vi "CmdExe.ExecCmd with Timeout and Abort_V2.vi"(0 "Working Dir":path=path "", 1 "Run minimized? (T)":bool=TRUE, 2 "Wait until completion? (T)":bool=TRUE, 3 "IgnoreStdErr":bool, 5 "Executable":string, 7 "StdIn":string, 9 "Arguements":string, 11 "error in":errorcluster, 12 "Timeout ms(-1)":i32=-1) -> (4 "STD OUT":string, 6 "STD ERR":string, 10 "Timed Out":bool, 13 "Aborted":bool, 14 "return code":i32, 15 "error out":errorcluster)   [LabVIEW 2024]
panel:
  out "Task Killed":bool
  # "Launch Cmd Exe"
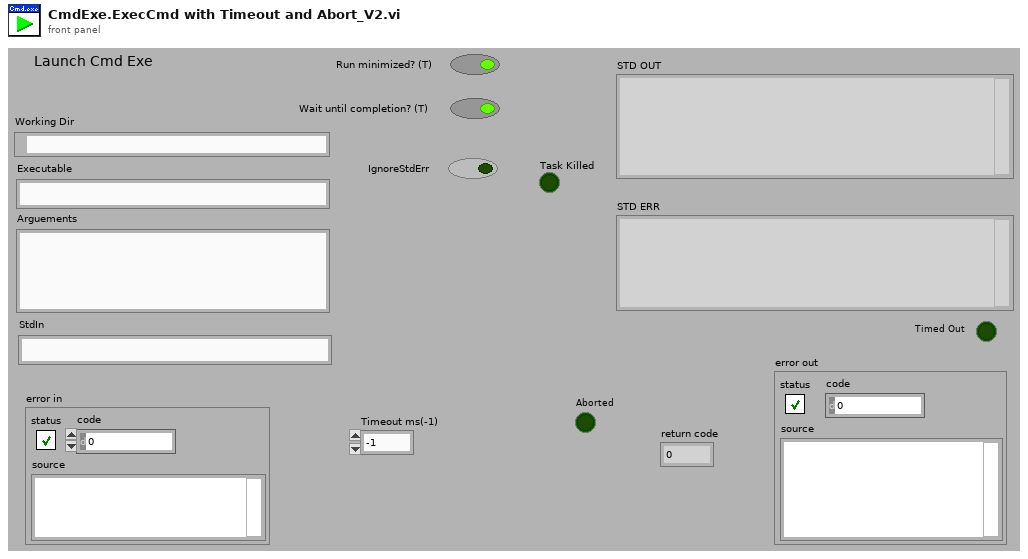
[diagram p1: front panel]
types:
  T1 = cluster{"Ref":refnum<vi>, "Abort":bool, "Timeout":bool, "Cmd":string, "Exe":string, "StdErr":string}
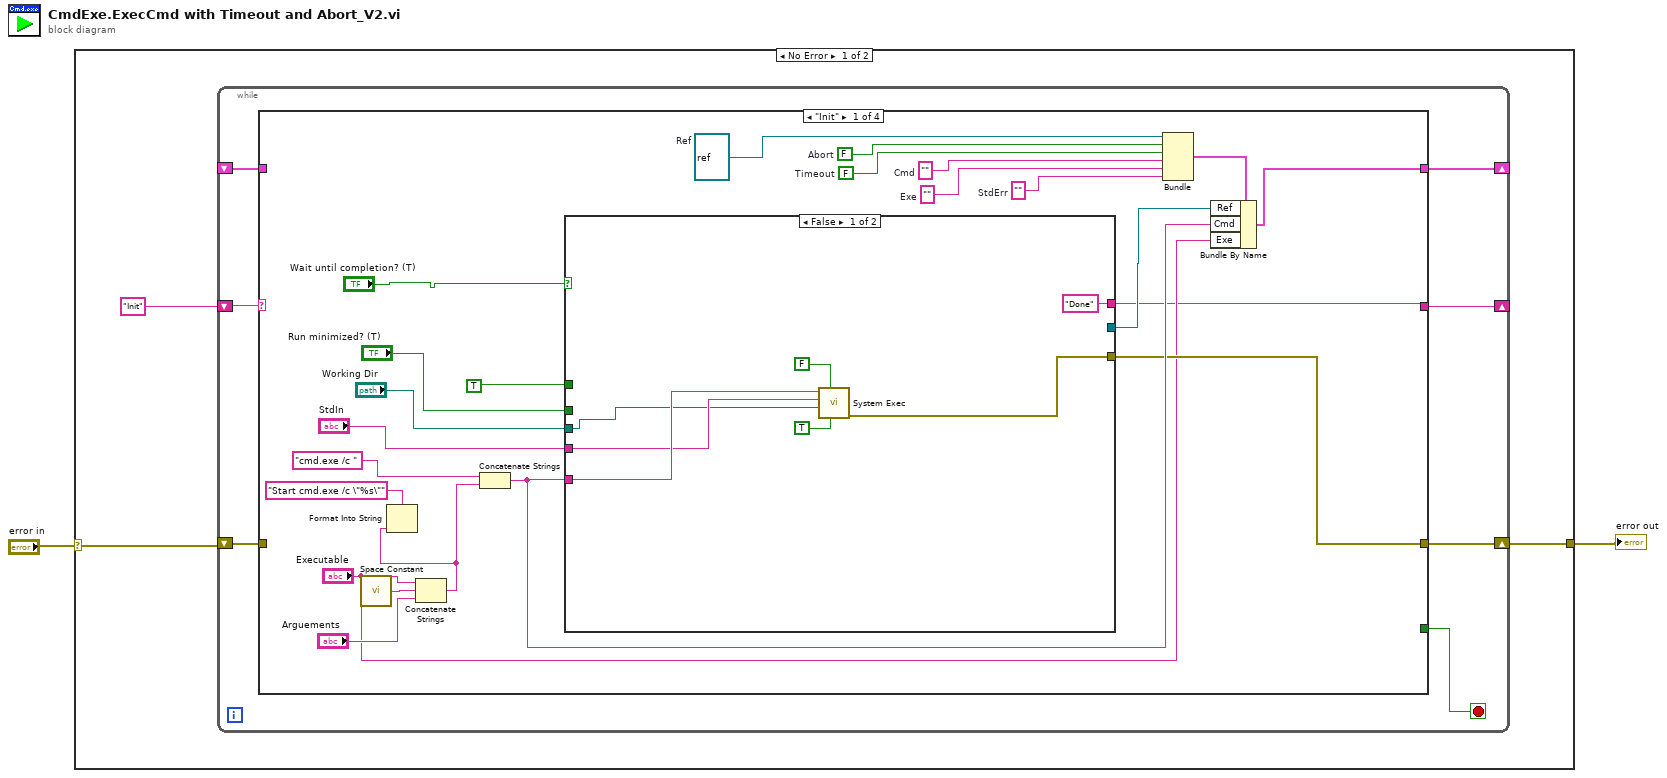
[diagram p0: block diagram]
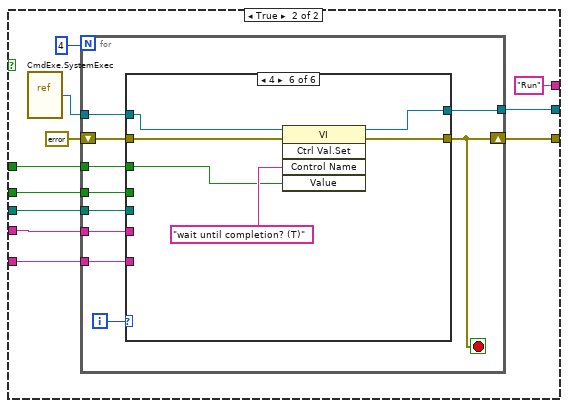
[diagram p2: hidden frame]
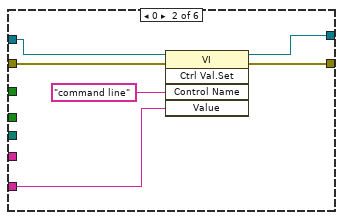
[diagram p4: hidden frame]
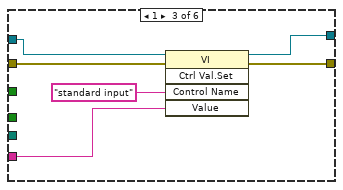
[diagram p5: hidden frame]
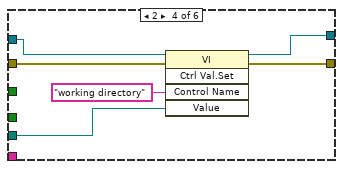
[diagram p6: hidden frame]
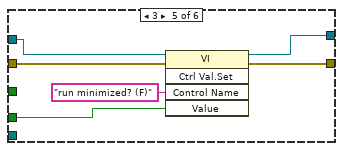
[diagram p7: hidden frame]
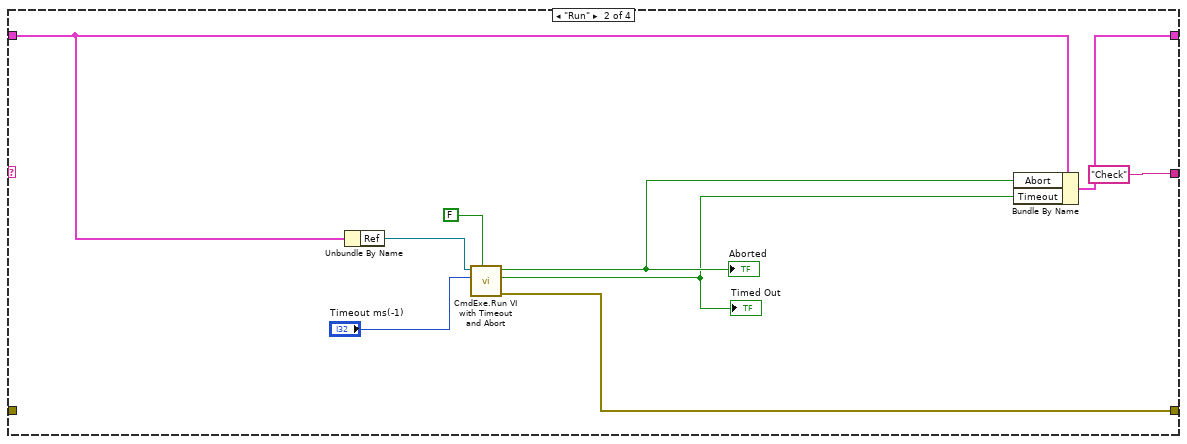
[diagram p8: hidden frame]
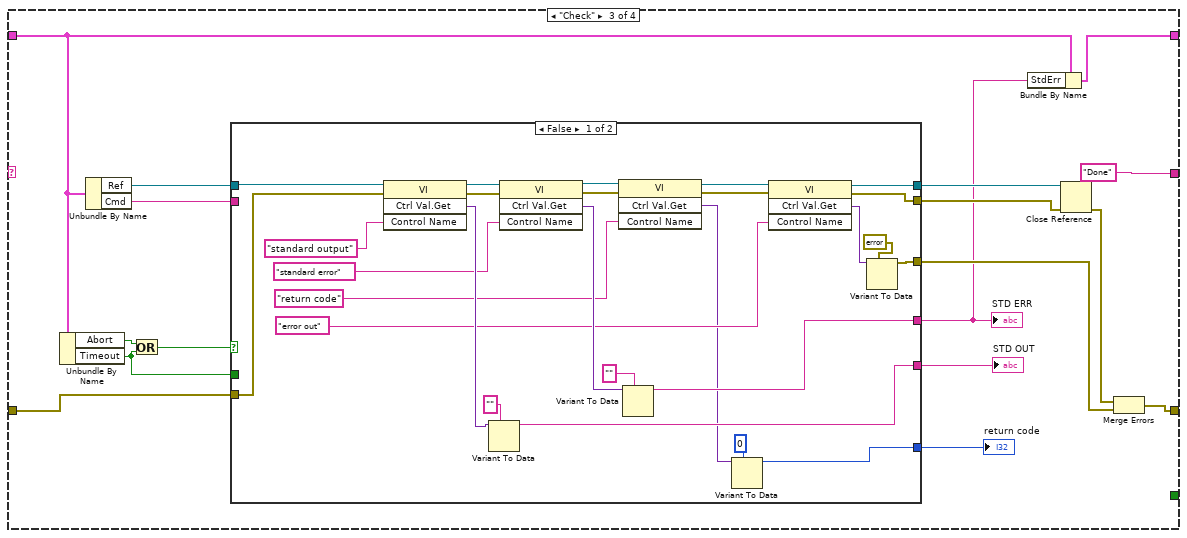
[diagram p9: hidden frame]
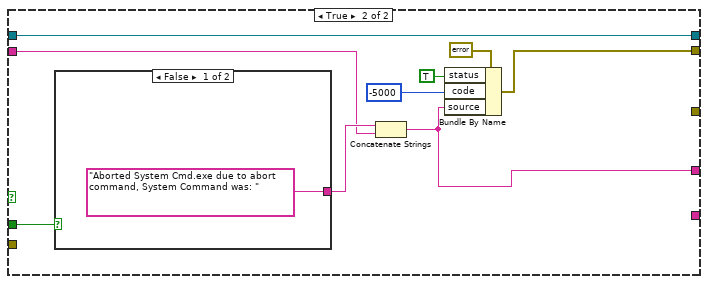
[diagram p10: hidden frame]
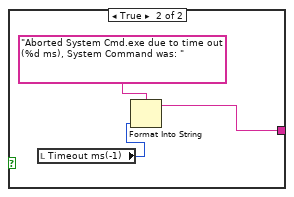
[diagram p11: hidden frame]
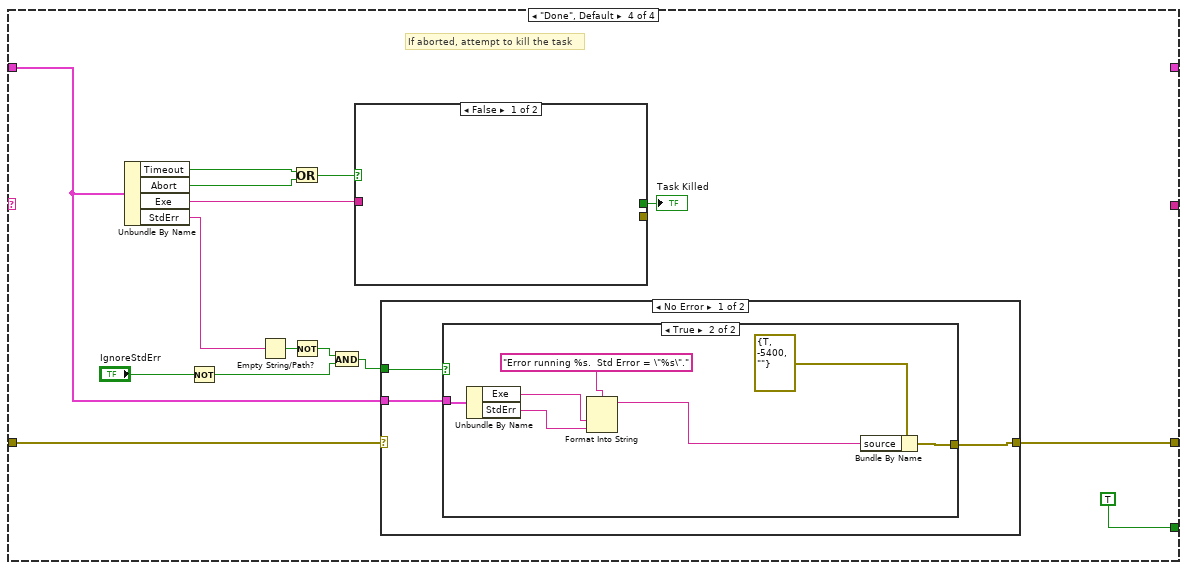
[diagram p12: hidden frame]
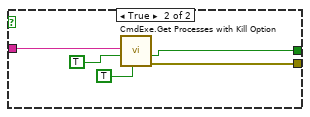
[diagram p15: hidden frame]
diagram:
  n1 = case shown="No Error" "error in" {
    selector: "error in" -> [w4 w192]
    tunnel: [w3 w192] -> w1
    frame No Error {
      n2 = while {
        shift-right: [w10] -> _
        shift-left: _ -> [w11]
        shift-right: [w9] -> _
        shift-left: "Init" -> [w12]
        shift-right: [w7] -> w3
        shift-left: w4 -> [w8]
        stop <- w6 stop-if-true
        n3 = case shown="\"Init\"" w12 {
          tunnel: w11 -> [_ w102 w108 w166]
          tunnel: [w29 w101 w107 _] -> w10
          tunnel: [w17 "Check" "Done" _] -> w9
          tunnel: [_ _ _ TRUE] -> w6
          tunnel: w8 -> [_ _ w113 w169]
          tunnel: [w24 w98 w111 w167] -> w7
          frame "Init" {
            w19 = ""  # StdErr
            w21 = ""  # Exe
            w26 = ""  # Cmd
            w27 = FALSE  # Timeout
            w28 = FALSE  # Abort
            w32 = refnum<vi> refnum  # Ref
            n4 = call <vilib>:"Space Constant.vi"() -> ("String"=w22:string)
            n5 = Concatenate Strings("Executable", w22, "Arguements") -> (w13:string)
            n6 = Format Into String(format string="Start cmd.exe /c \"%s\"", w13) -> ()  [unwired: 2 in, 2 out]
            n7 = Concatenate Strings("cmd.exe /c ", w13) -> (w25:string)
            n8 = case shown="False" "Wait until completion? (T)" {
              tunnel: "Run minimized? (T)" -> [_ w53]
              tunnel: "Working Dir" -> [w39 w52]
              tunnel: [_ w51] -> w31
              tunnel: w25 -> [w41 w50]
              tunnel: [w37 w49] -> w24
              tunnel: "StdIn" -> [w40 w48]
              tunnel: ["Done" "Run"] -> w17
              tunnel: TRUE -> [_ w43]
              frame False {
                n9 = call <vilib>:"System Exec.vi"("run minimized? (F)"=TRUE, "wait until completion? (T)"=FALSE, "working directory"=w39, "standard input"=w40, "command line"=w41) -> ("error out"=w37:errorcluster)  [unwired: 3 in, 3 out]
              }
              frame True {
                n10 = vi-ref "CmdExe.SystemExec.vi"() -> (w46:refnum<vi>)
                n11 = for {
                  N: 4 -> [_]
                  shift-right: [w54] -> w49
                  shift-left: errorcluster {"status"=FALSE, "code"=0, "source"=""} ("error constant") -> [w63]
                  tunnel: w46 -> [w62]
                  tunnel: [w61] -> w51
                  tunnel: w50 -> [w59]
                  tunnel: w48 -> [w58]
                  tunnel: w52 -> [w57]
                  tunnel: w53 -> [w56]
                  tunnel: w43 -> [w55]
                  i -> [w60]
                  stop <- w54 stop-if-true
                  n12 = case shown="4" w60 {
                    tunnel: w63 -> [w64 w70 w76 w82 w88 w94]
                    tunnel: w62 -> [w65 w69 w75 w81 w87 w93]
                    tunnel: [w64 w68 w74 w80 w86 w92] -> w54
                    tunnel: [w65 w67 w73 w79 w85 w91] -> w61
                    tunnel: w59 -> [_ w66 _ _ _ _]
                    tunnel: w58 -> [_ _ w72 _ _ _]
                    tunnel: w57 -> [_ _ _ w78 _ _]
                    tunnel: w56 -> [_ _ _ _ w84 _]
                    tunnel: w55 -> [_ _ _ _ _ w90]
                    frame 99, Default {
                    }
                    frame 0 {
                      n13 = invoke class="VI" method="Ctrl Val.Set"(reference=w69, error in=w70, "Control Name"="command line", "Value"=w66) -> (reference out=w67:refnum<vi>, error out=w68:errorcluster)  [unwired: 1 in, 3 out]
                    }
                    frame 1 {
                      n14 = invoke class="VI" method="Ctrl Val.Set"(reference=w75, error in=w76, "Control Name"="standard input", "Value"=w72) -> (reference out=w73:refnum<vi>, error out=w74:errorcluster)  [unwired: 1 in, 3 out]
                    }
                    frame 2 {
                      n15 = invoke class="VI" method="Ctrl Val.Set"(reference=w81, error in=w82, "Control Name"="working directory", "Value"=w78) -> (reference out=w79:refnum<vi>, error out=w80:errorcluster)  [unwired: 1 in, 3 out]
                    }
                    frame 3 {
                      n16 = invoke class="VI" method="Ctrl Val.Set"(reference=w87, error in=w88, "Control Name"="run minimized? (F)", "Value"=w84) -> (reference out=w85:refnum<vi>, error out=w86:errorcluster)  [unwired: 1 in, 3 out]
                    }
                    frame 4 {
                      n17 = invoke class="VI" method="Ctrl Val.Set"(reference=w93, error in=w94, "Control Name"="wait until completion? (T)", "Value"=w90) -> (reference out=w91:refnum<vi>, error out=w92:errorcluster)  [unwired: 1 in, 3 out]
                    }
                  }
                }
              }
            }
            n18 = Bundle("Ref"=w32, "Abort"=w28, "Timeout"=w27, "Cmd"=w26, "Exe"=w21, "StdErr"=w19) -> (w30:T1)  [unwired: 1 in]
            n19 = Bundle By Name(cluster=w30, "Ref"=w31, "Cmd"=w25, "Exe"="Executable") -> (w29:T1)
          }
          frame "Run" {
            n20 = Unbundle By Name(w102) -> ("Ref"=w97:refnum<vi>)
            n21 = call "CmdExe.Run VI with Timeout and Abort.vi"("Close Ref"=FALSE, "Timeout ms(-1)"="Timeout ms(-1)", "VI Refnum"=w97) -> ("error out"=w98:errorcluster, "Timeout"=w99:bool, "Abort"=w100:bool)  [unwired: 6 in]
            "Timed Out" <- w99
            "Aborted" <- w100
            n22 = Bundle By Name(cluster=w102, "Abort"=w100, "Timeout"=w99) -> (w101:T1)
          }
          frame "Check" {
            n23 = Unbundle By Name(w108) -> ("Abort"=w120:bool, "Timeout"=w114:bool)
            n24 = Unbundle By Name(w108) -> ("Ref"=w119:refnum<vi>, "Cmd"=w118:string)
            n25 = Or(x=w120, y=w114) -> (x .or. y?=w121:bool)
            n26 = case shown="False" w121 {
              tunnel: w119 -> [w147 w156]
              tunnel: [w135 w156] -> w116
              tunnel: [w134 w153] -> w115
              tunnel: [w138 w151] -> w106
              tunnel: [w137 _] -> w117
              tunnel: w118 -> [_ w149]
              tunnel: w114 -> [_ w148]
              tunnel: w113 -> [w136 _]
              tunnel: [w130 _] -> w110
              tunnel: [w122 _] -> w105
              frame False {
                n27 = invoke class="VI" method="Ctrl Val.Get"(reference=w147, error in=w136, "Control Name"="standard output") -> (reference out=w140:refnum<vi>, error out=w139:errorcluster, "Get Control Value Variant"=w145:variant)  [unwired: 1 in, 1 out]
                n28 = Variant To Data(type="", Variant=w145) -> (data=w137:string)  [unwired: 1 in, 1 out]
                n29 = invoke class="VI" method="Ctrl Val.Get"(reference=w140, error in=w139, "Control Name"="standard error") -> (reference out=w129:refnum<vi>, error out=w128:errorcluster, "Get Control Value Variant"=w142:variant)  [unwired: 1 in, 1 out]
                n30 = invoke class="VI" method="Ctrl Val.Get"(reference=w129, error in=w128, "Control Name"="return code") -> (reference out=w126:refnum<vi>, error out=w127:errorcluster, "Get Control Value Variant"=w124:variant)  [unwired: 1 in, 1 out]
                n31 = Variant To Data(type="", Variant=w142) -> (data=w138:string)  [unwired: 1 in, 1 out]
                n32 = Variant To Data(type=0 ("return code"), Variant=w124) -> (data=w122:i32)  [unwired: 1 in, 1 out]
                n33 = invoke class="VI" method="Ctrl Val.Get"(reference=w126, error in=w127, "Control Name"="error out") -> (reference out=w135:refnum<vi>, error out=w134:errorcluster, "Get Control Value Variant"=w132:variant)  [unwired: 1 in, 1 out]
                n34 = Variant To Data(type=errorcluster {"status"=FALSE, "code"=0, "source"=""} ("error constant"), Variant=w132) -> (data=w130:errorcluster)  [unwired: 1 in, 1 out]
              }
              frame True {
                n35 = case shown="False" w148 {
                  tunnel: ["Aborted System Cmd.exe due to abort command, System Command was: " ("source") w159] -> w152
                  frame False {
                  }
                  frame True {
                    n36 = local read "Timeout ms(-1)"() -> (w158:i32)
                    n37 = Format Into String(format string="Aborted System Cmd.exe due to time out (%d ms), System Command was: " ("source"), w158) -> (resulting string=w159:string)  [unwired: 2 in, 1 out]
                  }
                }
                n38 = Concatenate Strings(w152, w149) -> (w151:string)
                n39 = Bundle By Name(cluster=errorcluster {"status"=FALSE, "code"=0, "source"=""} ("error constant"), "status"=TRUE ("Wait Until Done"), "code"=-5000, "source"=w151) -> (w153:errorcluster)
              }
            }
            "STD ERR" <- w106
            "STD OUT" <- w117
            "return code" <- w105
            n40 = Bundle By Name(cluster=w108, "StdErr"=w106) -> (w107:T1)
            n41 = Close Reference(reference=w116, error in (no error)=w115) -> (error out=w112:errorcluster)
            n42 = Merge Errors(w112, w110) -> (w111:errorcluster)
          }
          frame "Done", Default {
            # "If aborted, attempt to kill the task"
            n43 = Unbundle By Name(w166) -> ("Timeout"=w173:bool, "Abort"=w172:bool, "Exe"=w174:string, "StdErr"=w168:string)
            n44 = Not(x="IgnoreStdErr") -> (.not. x?=w162:bool)
            n45 = Empty String/Path?(string/path=w168) -> (empty?=w164:bool)
            n46 = Or(x=w173, y=w172) -> (x .or. y?=w171:bool)
            n47 = Not(x=w164) -> (.not. x?=w161:bool)
            n48 = And(x=w161, y=w162) -> (x .and. y?=w165:bool)
            n49 = case shown="False" w171 {
              tunnel: w174 -> [_ w191]
              tunnel: [_ w188] -> _
              tunnel: [_ w187] -> w170
              frame False {
              }
              frame True {
                n50 = call "CmdExe.Get Processes with Kill Option.vi"("Kill Only 1 Instance"=TRUE, "Kill Task"=TRUE, "Process Name"=w191) -> ("Error Out"=w188:errorcluster, "Task Killed"=w187:bool)  [unwired: 5 in, 2 out]
              }
            }
            "Task Killed" <- w170
            n51 = case shown="No Error" w169 {
              selector: w169 -> [_ w186]
              tunnel: w165 -> [w178 _]
              tunnel: [w176 w186] -> w167
              tunnel: w166 -> [w177 _]
              frame No Error {
                n52 = case shown="True" w178 {
                  tunnel: w177 -> [_ w185]
                  tunnel: [_ w179] -> w176
                  frame False {
                    # "No error"
                  }
                  frame True {
                    n53 = Unbundle By Name(w185) -> ("Exe"=w182:string, "StdErr"=w181:string)
                    n54 = Format Into String(format string="Error running %s.  Std Error = \"%s\".", w182, w181) -> (resulting string=w180:string)  [unwired: 2 in, 1 out]
                    n55 = Bundle By Name(cluster=errorcluster {"status"=TRUE, "code"=-5400, "source"=""} ("error constant"), "source"=w180) -> (w179:errorcluster)
                  }
                }
              }
              frame Error {
              }
            }
          }
        }
      }
    }
    frame Error {
    }
  }
  "error out" <- w1
